vi "Ramp PSU to Target.vi"(6 "Axis":T1, 8 "error in (no error)":errorcluster, 9 "Target Rate (T/min)":dbl, 10 "Target Field (T)":dbl, 11 "Instrument.OxfordVRM in":refnum<class "Instrument.OxfordVRM.lvclass">) -> (0 "error out":errorcluster, 3 "Instrument.OxfordVRM out":refnum<class "Instrument.OxfordVRM.lvclass">)   [LabVIEW 2019, in "Instrument.OxfordVRM.lvclass"]
uses:
  Instrument.OxfordVRM.lvclass
  <userlib>/LevyLab/Levylab Instruments/Instrument Types/Cryostat/Typedefs/Magnet Axis--Enum.ctl
  <instrlib>/Mercury iXX/Public/Libraries/Magnet/Controls/PSU Actions.ctl
  <instrlib>/Mercury iXX/Public/Libraries/Magnet.lvlib
  <userlib>/LevyLab/Levylab Instruments/Instrument Types/Cryostat/Instrument.Cryostat.lvclass
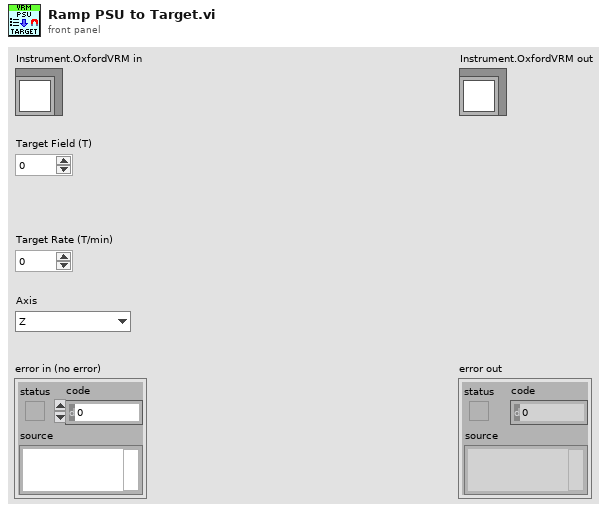
[diagram p1: front panel]
types:
  T1 = typedef "Instrument.Cryostat.lvclass/Magnet Axis--Enum.ctl" = enum16{"Z", "X", "Y"}
  T2 = typedef "Mercury iXX.lvlib/Magnet.lvlib/PSU Actions.ctl" = string
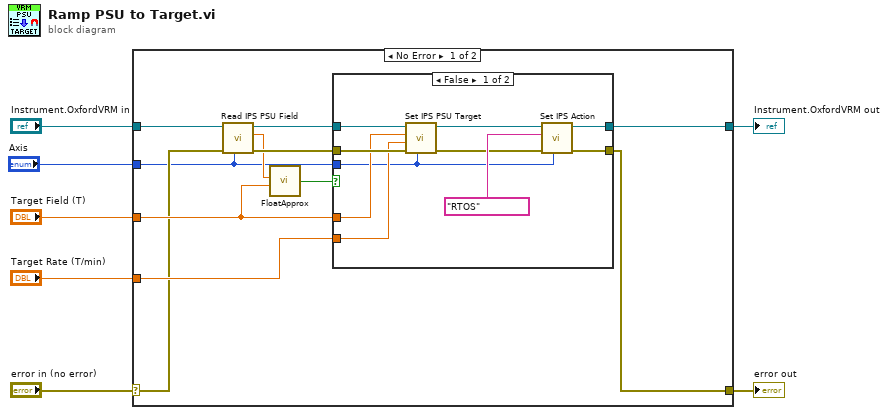
[diagram p0: block diagram]
diagram:
  n1 = case shown="No Error" "error in (no error)" {
    selector: "error in (no error)" -> [w11 w32]
    tunnel: [w14 w32] -> w6
    tunnel: [w18 w31] -> w4
    tunnel: "Instrument.OxfordVRM in" -> [w13 w31]
    tunnel: "Target Field (T)" -> [w16 _]
    tunnel: "Target Rate (T/min)" -> [w15 _]
    tunnel: "Axis" -> [w8 _]
    frame No Error {
      n2 = call "Read IPS PSU Field.vi"("Axis"=w8, "error in (no error)"=w11, "Instrument.OxfordVRM in"=w13) -> ("error out"=w10:errorcluster, "Power Supply Field (T)"=w9:dbl, "Instrument.OxfordVRM out"=w12:refnum<class "Instrument.OxfordVRM.lvclass">)  [unwired: 6 in]
      n3 = call "FloatApprox.vi"("y"=w16, "x"=w9) -> ("x ~ y?"=w17:bool)  [unwired: 4 in]
      n4 = case shown="False" w17 {
        tunnel: [w28 w30] -> w18
        tunnel: [w27 w29] -> w14
        tunnel: w12 -> [w25 w30]
        tunnel: w10 -> [w23 w29]
        tunnel: w16 -> [w20 _]
        tunnel: w15 -> [w21 _]
        tunnel: w8 -> [w19 _]
        frame False {
          n5 = call "Set IPS PSU Target.vi"("Axis"=w19, "error in (no error)"=w23, "Target Field Rate (T/min)"=w21, "Target Field (T)"=w20, "Instrument.OxfordVRM in"=w25) -> ("error out"=w22:errorcluster, "Instrument.OxfordVRM out"=w24:refnum<class "Instrument.OxfordVRM.lvclass">)  [unwired: 4 in, 1 out]
          n6 = call "Set IPS Action.vi"("Axis"=w19, "error in (no error)"=w22, "PSU Act Stat"=T2 "RTOS", "Instrument.OxfordVRM in"=w24) -> ("error out"=w27:errorcluster, "Instrument.OxfordVRM out"=w28:refnum<class "Instrument.OxfordVRM.lvclass">)  [unwired: 5 in, 1 out]
        }
        frame True {
          # "If PSU Field == Target, do nothing"
        }
      }
    }
    frame Error {
    }
  }
  "error out" <- w6
  "Instrument.OxfordVRM out" <- w4
